vi "Read Single Thermocouple.vi"(11 "Packet Data":u8[](array[numeric])) -> (3 "TC Data":T1)   [LabVIEW 2015]
uses:
  Thermocouple Data.ctl
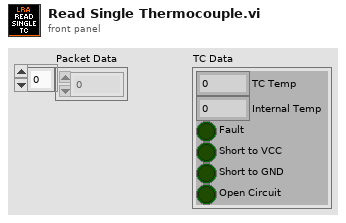
[diagram p1: front panel]
types:
  T1 = typedef "Thermocouple Data.ctl" = cluster{"TC Temp":dbl, "Internal Temp":dbl, "Fault":bool, "Short to VCC":bool, "Short to GND":bool, "Open Circuit":bool}
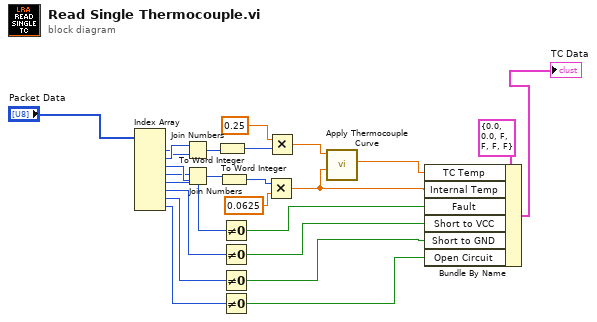
[diagram p0: block diagram]
diagram:
  n1 = Index Array(array="Packet Data") -> (element #1=w6:u8, element #2=w7:u8, element #3=w9:u8, element #4=w8:u8, element #5=w16:u8, element #6=w17:u8, element #7=w18:u8, element #8=w19:u8)  [unwired: 8 in]
  n2 = Join Numbers(hi=w7, lo=w6) -> ((hi.lo)=w10:u16)
  n3 = Join Numbers(hi=w8, lo=w9) -> ((hi.lo)=w11:u16)
  n4 = To Word Integer(number=w10) -> (16bit integer=w12:i16)
  n5 = To Word Integer(number=w11) -> (16bit integer=w13:i16)
  n6 = Not Equal To 0?(x=w16) -> (x != 0?=w20:bool)
  n7 = Not Equal To 0?(x=w17) -> (x != 0?=w21:bool)
  n8 = Not Equal To 0?(x=w18) -> (x != 0?=w22:bool)
  n9 = Not Equal To 0?(x=w19) -> (x != 0?=w23:bool)
  n10 = Multiply(x=w13, y=0.0625) -> (x*y=w1:dbl)
  n11 = Multiply(x=0.25, y=w12) -> (x*y=w3:dbl)
  n12 = call "Apply Thermocouple Curve.vi"("Internal Temp (°C)"=w1, "TC Reading (°C)"=w3) -> ("TC Out (°C)"=w2:dbl)  [unwired: 9 in]
  n13 = Bundle By Name(cluster=T1 {"TC Temp"=0.0, "Internal Temp"=0.0, "Fault"=FALSE, "Short to VCC"=FALSE, "Short to GND"=FALSE, "Open Circuit"=FALSE} ("TC Data"), "TC Temp"=w2, "Internal Temp"=w1, "Fault"=w20, "Short to VCC"=w21, "Short to GND"=w22, "Open Circuit"=w23) -> (→"TC Data":T1)
